vi "分中.vi"(8 "error in (no error)":errorcluster caption="错误输入（无错误）", 11 "信号数据":dbl[][](array[numeric])) -> (0 "error out":errorcluster caption="错误输出", 2 "分中角度":dbl)   [LabVIEW 2015, in "Logging.lvlib"]
uses:
  Logging.lvlib
panel:
  in  "取消按钮":bool
  in  "确定按钮":bool
  # "分中测量结果"
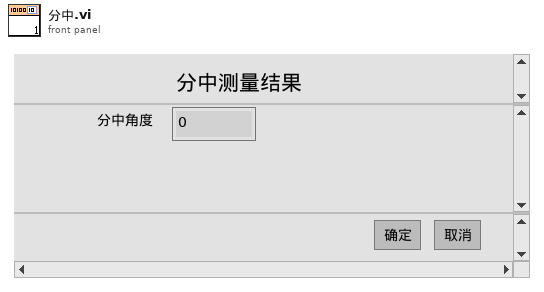
[diagram p1: front panel]
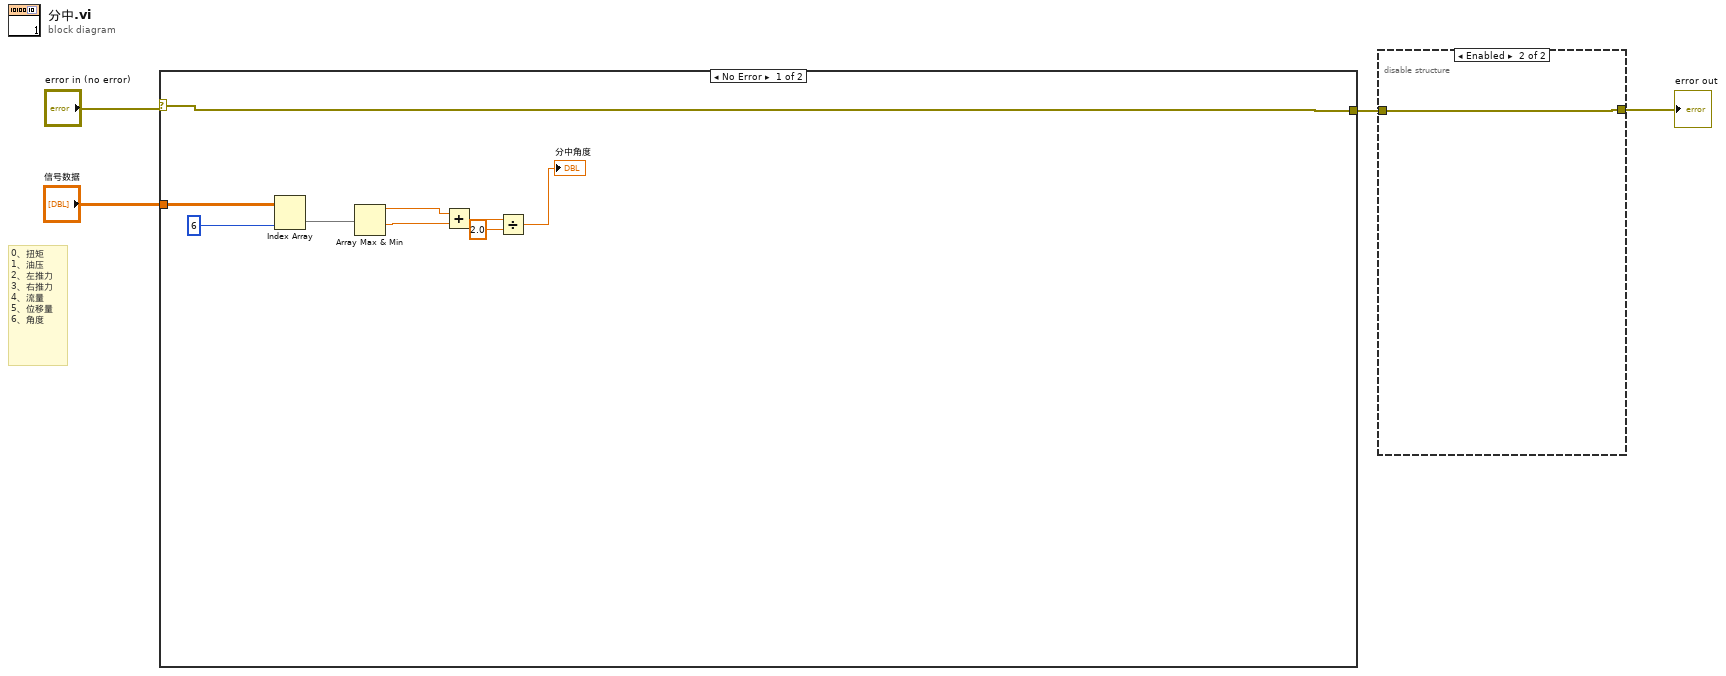
[diagram p0: block diagram]
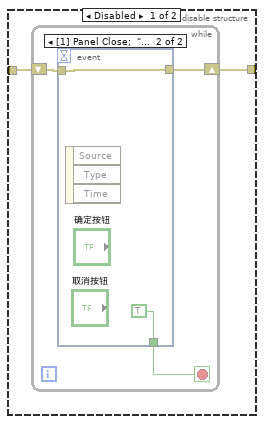
[diagram p2: hidden frame]
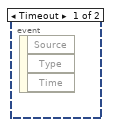
[diagram p3: hidden frame]
diagram:
  # "0、扭矩\n1、油压\n2、左推力\n3、右推力\n4、流量\n5、位移量\n6、角度"
  n1 = case shown="No Error" "error in (no error)" {
    selector: "error in (no error)" -> [w12 w14]
    tunnel: "信号数据" -> [w13 _]
    tunnel: [w12 w14] -> w1
    frame No Error {
      n2 = Index Array(array=w13, index (col)=6 ("禁用的索引 (列)")) -> (element=w10:dbl[])  [unwired: 1 in]
      n3 = Array Max & Min(array=w10) -> (max value=w9:dbl, min value=w8:dbl)  [unwired: 2 out]
      n4 = Add(x=w9, y=w8) -> (x+y=w7:dbl)
      n5 = Divide(x=w7, y=2.0) -> (x/y=→"分中角度":dbl)
    }
    frame Error {
    }
  }
  n6 = disable-structure shown="Enabled" {
    disable-tunnel: [w16 w22] -> w2
    disable-tunnel: w1 -> [w15 w22]
    frame Disabled {
      n7 = while {
        shift-right: [w19] -> w16
        shift-left: w15 -> [w18]
        stop <- w17 stop-if-true
        n8 = event shown="[1] Panel Close;  \"确定按钮\", \"取消按钮\": Value Change" {
          selector: _ -> [_ _]
          dyn-events: _ -> [_ _]
          timeout: _ -> [_ _]
          tunnel: [_ w21] -> w19
          tunnel: w18 -> [_ w21]
          tunnel: [_ TRUE] -> w17
          event Timeout {
            n9 = event-data() -> ()  [unwired: 1 in, 3 out]
          }
          event Panel Close; "确定按钮", "取消按钮": Value Change {
            n10 = event-data() -> ()  [unwired: 1 in, 3 out]
          }
        }
      }
    }
    frame Enabled {
    }
  }
  "error out" <- w2
